vi "FUG_MagnetPS.constructor.vi"(0 "name":string, 2 "data in":string, 5 "error in (no error)":errorcluster) -> (14 "i ref out":refnum<vi>, 16 "data out":string, 19 "error out":errorcluster)   [LabVIEW 2014, in "FUG_MagnetPS.lvlib"]
doc: "This is the constructor of a class.\n\nLicense Agreement for this software:\n\nCopyright (C)\nGesellschaft für Schwerionenforschung, GSI\nPlanckstr. 1\n64291 Darmstadt\nGermany\n\nContact: D.Beck@gsi.de \n\nThis program is free software; you can redistribute it and/or modify it under the terms of the GNU General Public License as published by the Free Software Foundation; either version 2 of the license, or (at your option) any later version.\n\nThis program is distributed in the hope that it will be useful, but WITHOUT ANY WARRANTY; without even the implied warranty of MERCHANTABILITY or FITNESS FOR A PARTICULAR PURPOSE. See the GNU General License for more details (http://www.gnu.org).\n\nGesellschaft für Schwerionenforschung, GSI\nPlanckstr. 1, 64291 Darmstadt, Germany\nFor all questions and ideas contact: M.Richter@gsi.de, H.Brand@gsi.de or D.Beck@gsi.de.\nLast update: 17-JUN-2004"
uses:
  FUG_MagnetPS.lvlib
  CSlibraries-extern/DimLVEvent/LVDimInterface/LVDimInterface.dim service type.ctl
  CS_Core/CSSystem/CSSystemLib/CSSystemLib.lvlib
  CS_Core/BaseProcess/BaseProcess.lvlib
  CSlibraries-extern/DimLVEvent/LVDimInterface/LVDimInterface.lvlib
  CS_PowerSupply/FUG_PowerSupply/FUG_PowerSupply.lvlib
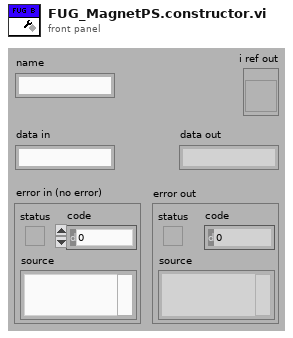
[diagram p1: front panel]
types:
  T1 = enum16{"SetAttribute", "GetAttribute", "CreateAttribute", "DestroyAttribute", "DestroyAllAtributes"}
  T2 = typedef "LVDimInterface.lvlib/LVDimInterface.dim service type.ctl" = u16
  T3 = typedef "BaseProcess.lvlib/BaseProcess.i attribute.ctl" = cluster{"EventStatus":string, "EventError":i32, "PresetEvtWatchD":i32, "PresetPdcWatchD":i32, "EventTimeout":i32, "PeriodicInterval":i32, "Interface":string[], "Address":string[], "Special":string[], "PeriodicError":i32, "PeriodicStatus":string, "SuperProc":string, "Descriptors":T4[], "CaseRef":refnum<vi>, "PdcRef":refnum<vi>, "Thread Ref":refnum<vi>, "eventErrorID":i32, "eventStatusID":i32, "periodicErrorID":i32, "periodicStatusID":i32, "pdcCtrID":i32}
  T4 = typedef "BaseProcess.lvlib/BaseProcess.descriptor definition.ctl" = cluster{"selector":string, "descriptor":T5}
  T5 = typedef "BaseProcess.lvlib/BaseProcess.descriptor string definition.ctl" = string
  T6 = typedef "FUG_MagnetPS.lvlib/FUG_MagnetPS.i attribute.ctl" = cluster{"Gaussmeter":string, "SetField":dbl, "MagneticField queue":refnum<queue>, "Field Callback ID":i32, "nomCurrent":dbl, "Proportional":dbl, "Regulation?":bool, "actFieldID":i32, "nomFieldID":i32, "nomAutoCurrentID":i32, "regCurrentID":i32}
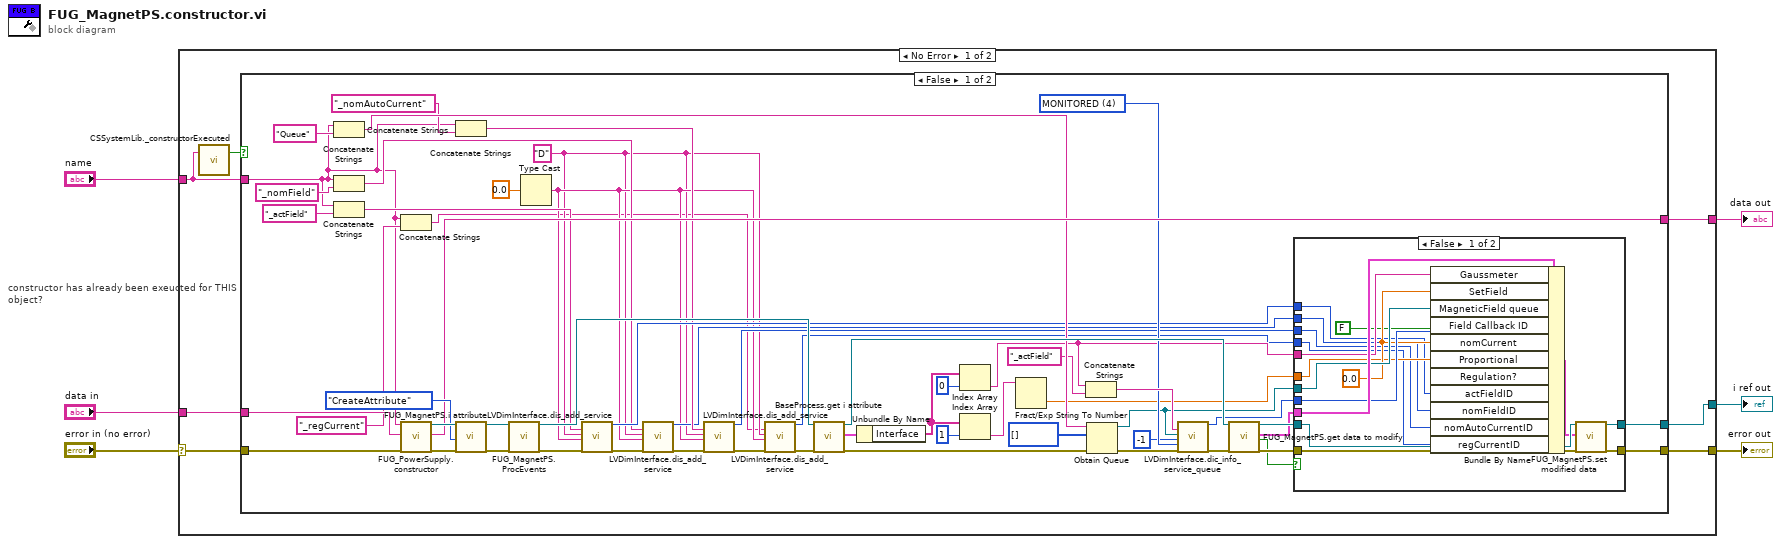
[diagram p0: block diagram]
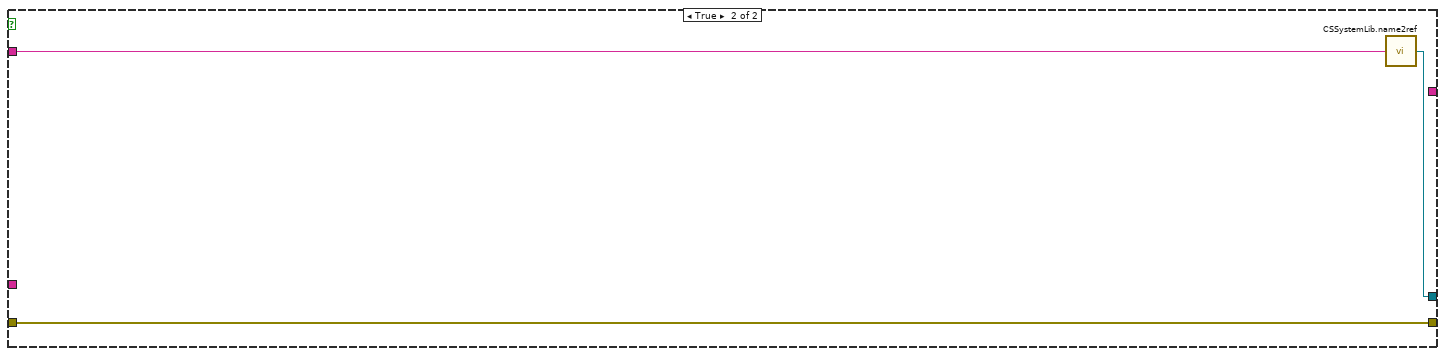
[diagram p3: hidden frame]
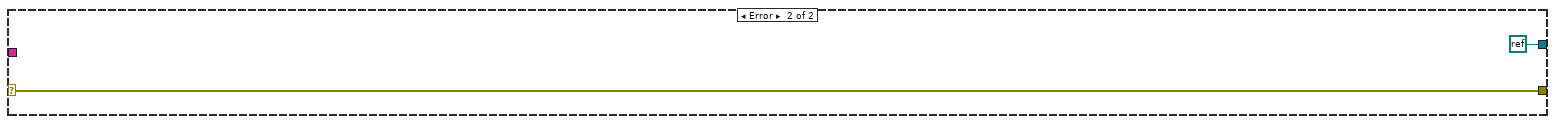
[diagram p4: hidden frame]
diagram:
  n1 = case shown="No Error" "error in (no error)" {
    selector: "error in (no error)" -> [w11 w91]
    tunnel: [w13 refnum<k0> refnum] -> w6
    tunnel: [w12 w91] -> w5
    tunnel: "name" -> [w9 _]
    tunnel: "data in" -> [w8 _]
    tunnel: [w7 _] -> w1
    frame No Error {
      n2 = call "CSSystemLib._constructorExecuted.vi"("name"=w9) -> ("constructor executed?"=w10:bool)  [unwired: 18 in]
      n3 = case "constructor has already been exeucted for THIS object?" shown="False" w10 {
        tunnel: [w56 w89] -> w13
        tunnel: [w55 w88] -> w12
        tunnel: w9 -> [w15 w90]
        tunnel: w11 -> [w66 w88]
        tunnel: w8 -> [w65 _]
        tunnel: [w64 _] -> w7
        frame False {
          w18 = "D" ("typeDescriptor")
          w49 = T2 4 items=["ONCE_ONLY"=1, "TIMED"=2, "MONITORED"=4] ("serviceType")
          n4 = Concatenate Strings(w15, "Queue" ("string")) -> (w54:string)
          n5 = Concatenate Strings(w15, "_nomField") -> (w26:string)
          n6 = Concatenate Strings(w15, "_actField") -> (w33:string)
          n7 = Concatenate Strings(w15, "_regCurrent") -> (w16:string)
          n8 = call "FUG_PowerSupply.constructor.vi"("name"=w15, "data in"=w65, "error in(no error)"=w66) -> ("i ref out"=w69:refnum<vi>, "data out"=w64:string, "error out"=w68:errorcluster)  [unwired: 14 in]
          n9 = Concatenate Strings(w15, "_nomAutoCurrent") -> (w24:string)
          n10 = call "FUG_MagnetPS.i attribute.vi"("VI Refnum"=w69, "Action"=T1."CreateAttribute", "error in (no error)"=w68) -> ("VI Refnum out"=w35:refnum<vi>, "error out"=w37:errorcluster)  [unwired: 14 in, 1 out]
          n11 = call "FUG_MagnetPS.ProcEvents.vi"("i ref in"=w35, "error in (no error)"=w37) -> ("i ref out"=w36:refnum<vi>, "error out"=w31:errorcluster)  [unwired: 16 in]
          n12 = Type Cast(x=0.0 ("D32")) -> (*(type *) &x=w19:string)  [unwired: 1 in]
          n13 = call "LVDimInterface.dis_add_service.vi"("serviceName"=w33, "typeDescriptor"=w18, "data"=w19, "error in (no error)"=w31) -> ("my_serviceID"=w30:i32, "error out"=w29:errorcluster)  [unwired: 14 in]
          n14 = call "LVDimInterface.dis_add_service.vi"("serviceName"=w26, "typeDescriptor"=w18, "data"=w19, "error in (no error)"=w29) -> ("my_serviceID"=w23:i32, "error out"=w28:errorcluster)  [unwired: 14 in]
          n15 = call "LVDimInterface.dis_add_service.vi"("serviceName"=w24, "typeDescriptor"=w18, "data"=w19, "error in (no error)"=w28) -> ("my_serviceID"=w22:i32, "error out"=w21:errorcluster)  [unwired: 14 in]
          n16 = call "LVDimInterface.dis_add_service.vi"("serviceName"=w16, "typeDescriptor"=w18, "data"=w19, "error in (no error)"=w21) -> ("my_serviceID"=w14:i32, "error out"=w20:errorcluster)  [unwired: 14 in]
          n17 = call "BaseProcess.get i attribute.vi"("i ref in"=w36, "error in (no error)"=w20) -> ("i ref out"=w59:refnum<vi>, "i attribute"=w58:T3, "error out"=w46:errorcluster)  [unwired: 15 in]
          n18 = Unbundle By Name(w58) -> ("Interface"=w41:string[])
          n19 = Index Array(array=w41, index=0) -> (element=w43:string)
          n20 = Index Array(array=w41, index=1) -> (element=w39:string)
          n21 = Fract/Exp String To Number(string=w39) -> (number=w38:dbl)  [unwired: 3 in, 1 out]
          n22 = Concatenate Strings(w43, "_actField" ("string")) -> (w50:string)
          n23 = Obtain Queue(name (unnamed)=w54, element data type=i8[] [], error in (no error)=w46) -> (queue out=w44:refnum<queue>, error out=w51:errorcluster)  [unwired: 2 in, 1 out]
          n24 = call "LVDimInterface.dic_info_service_queue.vi"("serviceName"=w50, "queueRef"=w44, "timeout [s]"=-1, "serviceType"=w49, "error in (no error)"=w51) -> ("callBackID"=w45:i32, "error out"=w47:errorcluster)  [unwired: 13 in]
          n25 = call "FUG_MagnetPS.get data to modify.vi"("i ref in"=w59, "error in (no error)"=w47) -> ("i ref out"=w63:refnum<vi>, "i attribute"=w61:T6, "timed out"=w60:bool, "error out"=w62:errorcluster)  [unwired: 14 in]
          n26 = case shown="False" w60 {
            tunnel: w63 -> [w85 w87]
            tunnel: [w84 w87] -> w56
            tunnel: w62 -> [w83 w86]
            tunnel: [w82 w86] -> w55
            tunnel: w61 -> [w81 _]
            tunnel: w43 -> [w79 _]
            tunnel: w45 -> [w78 _]
            tunnel: w44 -> [w77 _]
            tunnel: w38 -> [w75 _]
            tunnel: w30 -> [w73 _]
            tunnel: w23 -> [w72 _]
            tunnel: w22 -> [w71 _]
            tunnel: w14 -> [w70 _]
            frame False {
              w76 = 0.0 ("SetField")
              n27 = Bundle By Name(cluster=w81, "Gaussmeter"=w79, "SetField"=w76, "MagneticField queue"=w77, "Field Callback ID"=w78, "nomCurrent"=w76, "Proportional"=w75, "Regulation?"=FALSE, "actFieldID"=w73, "nomFieldID"=w72, "nomAutoCurrentID"=w71, "regCurrentID"=w70) -> (w80:T6)
              n28 = call "FUG_MagnetPS.set modified data.vi"("i ref in"=w85, "i attribute"=w80, "error in (no error)"=w83) -> ("i ref out"=w84:refnum<vi>, "error out"=w82:errorcluster)  [unwired: 15 in]
            }
            frame True {
            }
          }
        }
        frame True {
          n29 = call "CSSystemLib.name2ref.vi"("name"=w90) -> ("obj refnum"=w89:refnum<vi>)
        }
      }
    }
    frame Error {
    }
  }
  "i ref out" <- w6
  "error out" <- w5
  "data out" <- w1
